vi "QI_ConfigCam_old.vi"(4 "CCD Height":u32, 6 "CCD Width":u32, 7 "path to dll":path, 8 "error in (no error)":errorcluster, 9 "paramVal":u32, 10 "Parameter":T1, 11 "Camera Handle":u32) -> (0 "error out":errorcluster, 1 "ConfigCam err":i32, 3 "Camera Handle":u32)   [LabVIEW 2014]
uses:
  Controls/Parameter.ctl
  Release/QImaging.dll
panel:
  in  "paramKey":u32
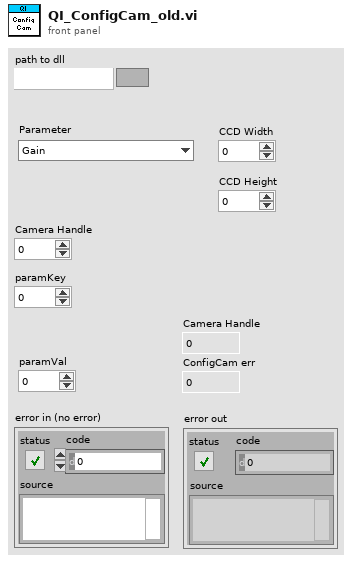
[diagram p1: front panel]
types:
  T1 = typedef "Parameter.ctl" = enum32{"Gain ", "Offset", "Exposure", "Binning", "HzBinning", "VtBinning", "Readout speed", "Trigger Type", "Color Wheel", "Cooler Active", "Exposure red", "Exposure blue", "Image format", "ROI X", "ROI Y", "ROI Width", "ROI Height"}
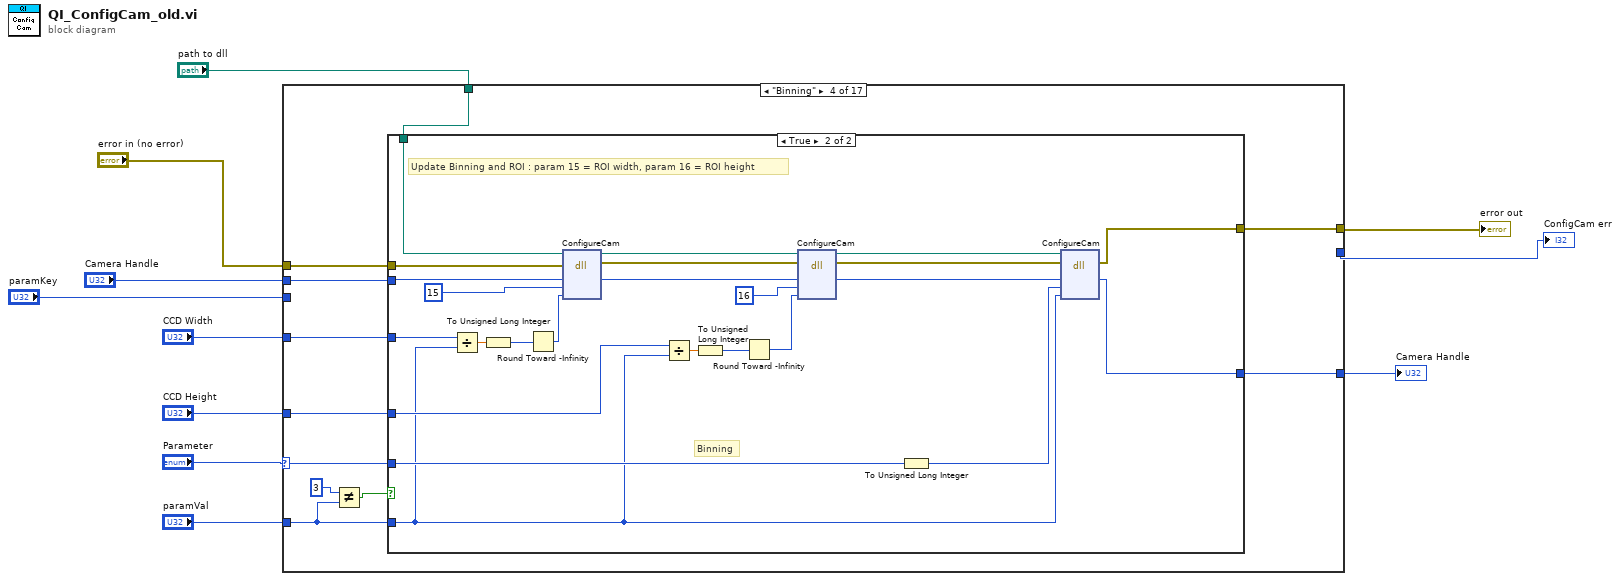
[diagram p0: block diagram]
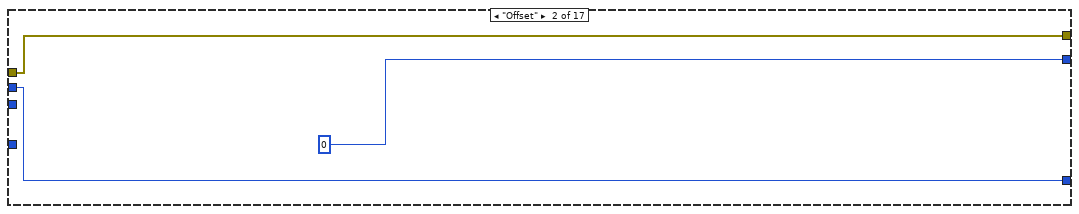
[diagram p3: hidden frame]
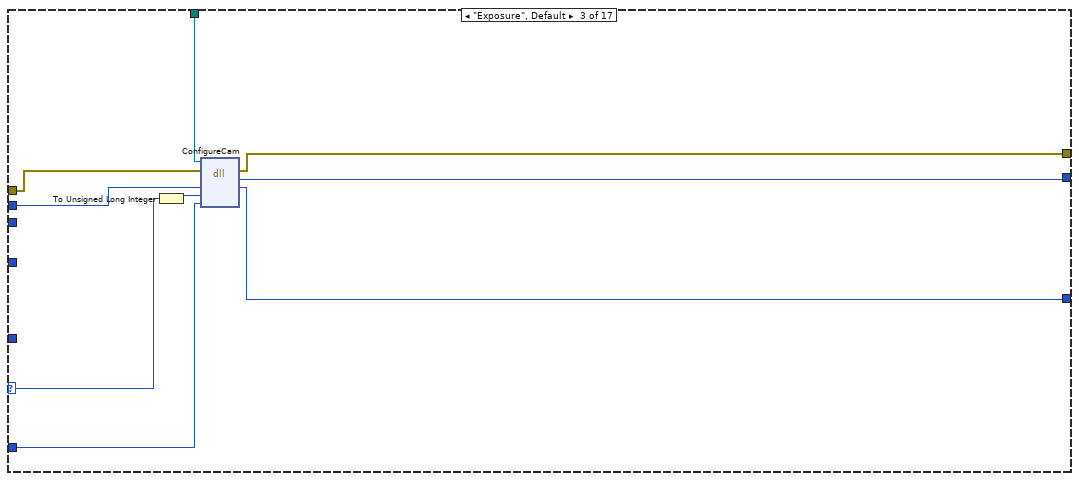
[diagram p4: hidden frame]
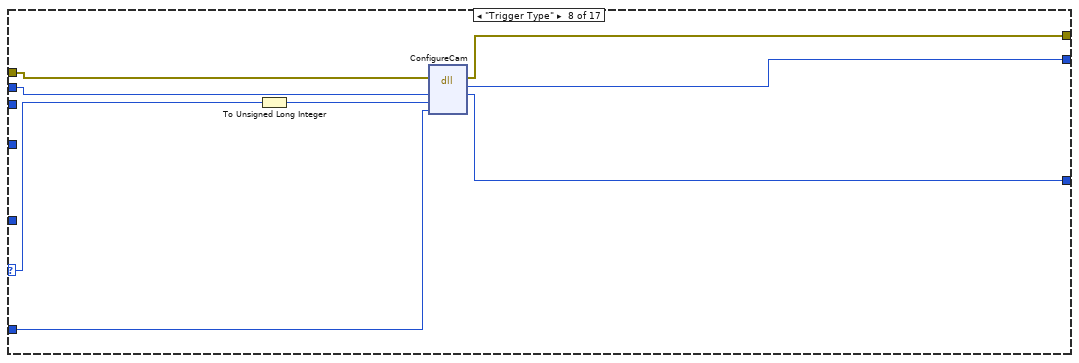
[diagram p9: hidden frame]
diagram:
  n1 = case shown="\"Binning\"" "Parameter" {
    selector: "Parameter" -> [_ _ w20 w30 _ _ _ w71 _ _ _ _ _ _ _ _ _]
    tunnel: "error in (no error)" -> [w13 w16 w25 w35 w64 w66 w67 w76 w78 w80 w82 w84 w86 w88 w90 w92 w94]
    tunnel: [w13 w16 w23 w34 w64 w66 w67 w75 w78 w80 w82 w84 w86 w88 w90 w92 w94] -> w10
    tunnel: "Camera Handle" -> [w12 w15 w24 w36 w63 w65 w68 w74 w77 w79 w81 w83 w85 w87 w89 w91 w93]
    tunnel: "paramVal" -> [_ _ w22 w33 _ _ _ w70 _ _ _ _ _ _ _ _ _]
    tunnel: "paramKey" -> [_ _ _ _ _ _ _ _ _ _ _ _ _ _ _ _ _]
    tunnel: [w12 w15 w19 w27 w63 w65 w68 w73 w77 w79 w81 w83 w85 w87 w89 w91 w93] -> w5
    tunnel: [_ 0 w18 _ _ _ _ w72 _ _ _ _ _ _ _ _ _] -> w4
    tunnel: "CCD Width" -> [_ _ _ w29 _ _ _ _ _ _ _ _ _ _ _ _ _]
    tunnel: "CCD Height" -> [_ _ _ w28 _ _ _ _ _ _ _ _ _ _ _ _ _]
    tunnel: "path to dll" -> [_ _ w17 w26 _ _ _ _ _ _ _ _ _ _ _ _ _]
    frame "Gain " {
    }
    frame "Offset" {
    }
    frame "Exposure", Default {
      n2 = To Unsigned Long Integer(number=w20) -> (unsigned 32bit integer=w21:u32)
      n3 = dll-call lib="C:/Users/appli/Documents/Aline/octo-labview/QImaging/Release/QImaging.dll" fn="ConfigureCam"(path in=w17, error in=w25, "handle"=w24, "paramKey"=w21, "paramVal"=w22) -> (error out=w23:errorcluster, "return type"=w18:i32, "handle"=w19:u32)  [unwired: 3 in, 1 out]
    }
    frame "Binning" {
      n4 = Not Equal?(x=u32 3, y=w33) -> (x != y?=w31:bool)
      n5 = case shown="True" w31 {
        tunnel: w36 -> [w37 w62]
        tunnel: w35 -> [w38 w61]
        tunnel: w33 -> [_ w46]
        tunnel: [w38 w58] -> w34
        tunnel: w30 -> [_ w49]
        tunnel: w29 -> [_ w53]
        tunnel: w28 -> [_ w50]
        tunnel: [w37 w47] -> w27
        tunnel: w26 -> [_ w41]
        frame False {
        }
        frame True {
          # "Binning"
          # "Update Binning and ROI : param 15 = ROI width, param 16 = ROI height"
          n6 = Divide(x=w53, y=w46) -> (x/y=w52:dbl)
          n7 = To Unsigned Long Integer(number=w52) -> (unsigned 32bit integer=w43:u32)
          n8 = Round Toward -Infinity(1:w43) -> (0:w42:u32)
          n9 = dll-call lib="C:/Users/appli/Documents/Aline/octo-labview/QImaging/Release/QImaging.dll" fn="ConfigureCam"(path in=w41, error in=w61, "handle"=w62, "paramKey"=u32 15, "paramVal"=w42) -> (path out=w40:path, error out=w60:errorcluster, "handle"=w55:u32)  [unwired: 4 in]
          n10 = Divide(x=w50, y=w46) -> (x/y=w51:dbl)
          n11 = To Unsigned Long Integer(number=w51) -> (unsigned 32bit integer=w45:u32)
          n12 = Round Toward -Infinity(1:w45) -> (0:w44:u32)
          n13 = dll-call lib="C:/Users/appli/Documents/Aline/octo-labview/QImaging/Release/QImaging.dll" fn="ConfigureCam"(path in=w40, error in=w60, "handle"=w55, "paramKey"=u32 16, "paramVal"=w44) -> (path out=w39:path, error out=w59:errorcluster, "handle"=w56:u32)  [unwired: 4 in]
          n14 = To Unsigned Long Integer(number=w49) -> (unsigned 32bit integer=w57:u32)
          n15 = dll-call lib="C:/Users/appli/Documents/Aline/octo-labview/QImaging/Release/QImaging.dll" fn="ConfigureCam"(path in=w39, error in=w59, "handle"=w56, "paramKey"=w57, "paramVal"=w46) -> (error out=w58:errorcluster, "handle"=w47:u32)  [unwired: 4 in, 1 out]
        }
      }
    }
    frame "HzBinning" {
    }
    frame "VtBinning" {
    }
    frame "Readout speed" {
    }
    frame "Trigger Type" {
      n16 = To Unsigned Long Integer(number=w71) -> (unsigned 32bit integer=w69:u32)
      n17 = dll-call lib="Z:/Programmes en Developpement/QImaging/Release/QImaging.dll" fn="ConfigureCam"(error in=w76, "handle"=w74, "paramKey"=w69, "paramVal"=w70) -> (error out=w75:errorcluster, "return type"=w72:i32, "handle"=w73:u32)  [unwired: 4 in, 1 out]
    }
    frame "Color Wheel" {
    }
    frame "Cooler Active" {
    }
    frame "Exposure red" {
    }
    frame "Exposure blue" {
    }
    frame "Image format" {
    }
    frame "ROI X" {
    }
    frame "ROI Y" {
    }
    frame "ROI Width" {
    }
    frame "ROI Height" {
    }
  }
  "error out" <- w10
  "Camera Handle" <- w5
  "ConfigCam err" <- w4
